vi "Error Dialog Reference Globals.vi"() -> (0 "Open?":refnum<vi>, 1 "Error in":refnum<vi>, 2 "VI reference":refnum<vi>)   [LabVIEW 2020, in "Multiple Errors.lvclass"]
uses:
  Multiple Errors.lvclass
  Dialog.vi
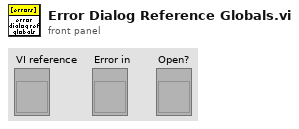
[diagram p1: front panel]
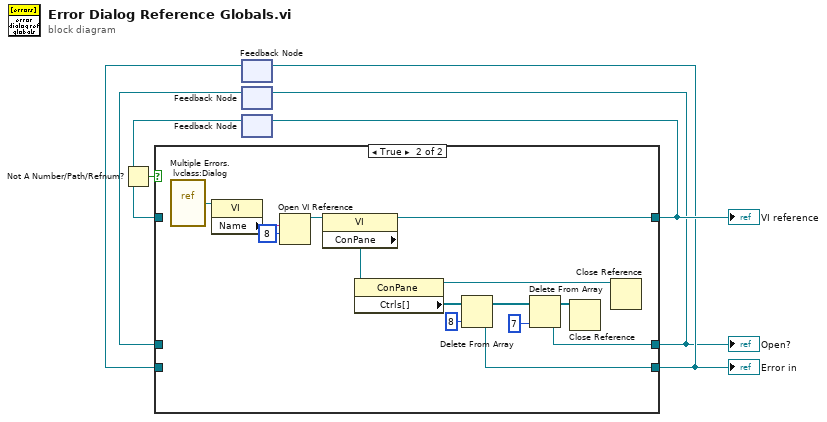
[diagram p0: block diagram]
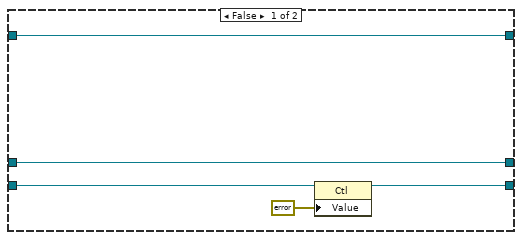
[diagram p2: hidden frame]
diagram:
  n1 = feedback #1() -> (w4:refnum<vi>)  [unwired: 1 in]
  n2 = feedback #2() -> (w1:refnum<vi>)  [unwired: 1 in]
  n3 = feedback #3() -> (w6:refnum<vi>)  [unwired: 1 in]
  n4 = Not A Number/Path/Refnum?(number/path/refnum=w6) -> (NaN/Path/Refnum?=w7:bool)
  n5 = case shown="True" w7 {
    tunnel: w6 -> [w12 _]
    tunnel: [w12 w18] -> w5
    tunnel: [w10 w17] -> w3
    tunnel: w4 -> [w11 _]
    tunnel: [w8 w13] -> w2
    tunnel: w1 -> [w8 _]
    frame False {
      n6 = property class="Ctl"(reference=w11, "Value"=errorcluster {"status"=FALSE, "code"=0, "source"=""} ("error in (no error)")) -> (reference out=w10:refnum<vi>)  [unwired: 1 in, 1 out]
    }
    frame True {
      n7 = vi-ref "Multiple Errors.lvclass:Dialog.vi"() -> (w22:refnum<vi>)
      n8 = property class="VI"(reference=w22) -> ("Name"=w21:string)  [unwired: 1 in, 2 out]
      n9 = Open VI Reference(vi path=w21, options=8) -> (vi reference=w19:refnum<vi>)  [unwired: 4 in, 1 out]
      n10 = property class="VI"(reference=w19) -> (reference out=w18:refnum<vi>, "ConPane"=w26:refnum<vi>)  [unwired: 1 in, 1 out]
      n11 = property class="ConPane"(reference=w26) -> (reference out=w23:refnum<vi>, "Ctrls[]"=w24:refnum<vi>[])  [unwired: 1 in, 1 out]
      n12 = Delete From Array(array=w24, index=8) -> (deleted portion=w17:refnum<vi>, array with subset deleted=w16:refnum<vi>[])  [unwired: 1 in]
      n13 = Delete From Array(array=w16, index=7) -> (deleted portion=w13:refnum<vi>, array with subset deleted=w15:refnum<vi>[])  [unwired: 1 in]
      n14 = Close Reference(reference=w15) -> ()  [unwired: 1 in, 1 out]
      n15 = Close Reference(reference=w23) -> ()  [unwired: 1 in, 1 out]
    }
  }
  "VI reference" <- w5
  "Error in" <- w3
  "Open?" <- w2
  n16 = feedback-in #1(w3) -> ()
  n17 = feedback-in #2(w2) -> ()
  n18 = feedback-in #3(w5) -> ()
